vi "testy2.vi"() -> ()   [LabVIEW 2021]
panel:
  out "size(s)":i32[](array[numeric])
  out "output array":dbl[][](array[numeric])
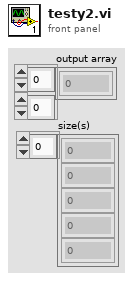
[diagram p1: front panel]
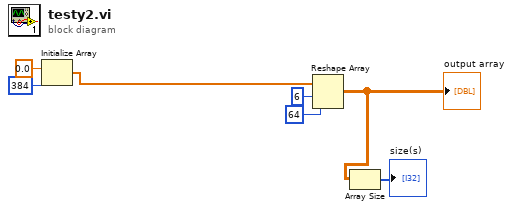
[diagram p0: block diagram]
diagram:
  n1 = Initialize Array(0.0 ("element"), 384 ("dimension size")) -> (w5:dbl[])
  n2 = Reshape Array(w5, 6 ("dimension size"), 64 ("dimension size")) -> (w2:dbl[][])
  "output array" <- w2
  n3 = Array Size(array=w2) -> (size(s)=→"size(s)":i32[])
